vi "Arm timer thinking.vi"(8 "error in":errorcluster, 11 "Philosopher in":refnum<class "Philosopher.lvclass">) -> (0 "error out":errorcluster, 3 "Philosopher out":refnum<class "Philosopher.lvclass">)   [LabVIEW 2021, in "Philosopher.lvclass"]
uses:
  Philosopher.lvclass
  Message Pump/Message Pump.lvclass
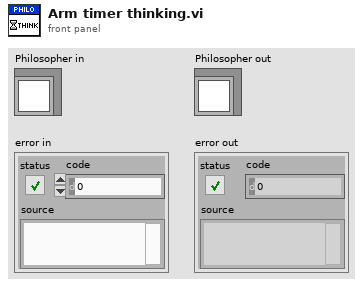
[diagram p1: front panel]
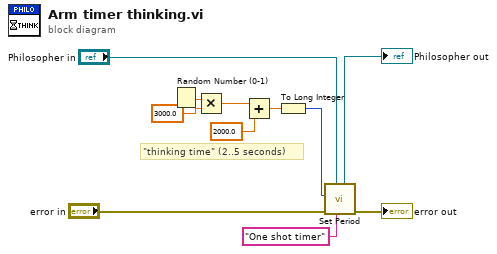
[diagram p0: block diagram]
diagram:
  # "\"thinking time\" (2..5 seconds)"
  n1 = Random Number (0-1)() -> (number: 0 to 1=w3:dbl)
  n2 = Multiply(x=w3, y=3000.0) -> (x*y=w2:dbl)
  n3 = Add(x=w2, y=2000.0) -> (x+y=w4:dbl)
  n4 = To Long Integer(number=w4) -> (32bit integer=w5:i32)
  n5 = call "Set Period.vi"("Worker Alias"="One shot timer", "Caller"="Philosopher in", "error in"="error in", "Period (ms)"=w5) -> ("error out"=→"error out":errorcluster, "dup Caller out"=→"Philosopher out":refnum<class "Philosopher.lvclass">)  [unwired: 6 in]
